vi "get Owner.vi"(11 "Deployable in":refnum<class "Deployable.lvclass">) -> (3 "Player":T1)   [LabVIEW 2021, in "Deployable.lvclass"]
uses:
  Deployable.lvclass
  Deployable.lvclass/Deployable.ctl
  Actors/Main Controller/Actor/Player.ctl
  Actors/Main Controller/Actor/Main Controller Actor.lvclass
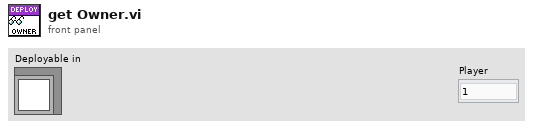
[diagram p1: front panel]
types:
  T1 = typedef "Main Controller Actor.lvclass/Player.ctl" = enum16{"1", "2"}
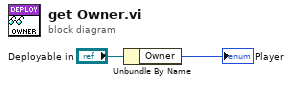
[diagram p0: block diagram]
diagram:
  n1 = Unbundle By Name("Deployable in") -> ("Owner"=→"Player":T1)
